vi "testTwoServersReportLogMessages.vi"(8 "error in":errorcluster) -> (0 "error out":errorcluster)   [LabVIEW 2018]
uses:
  <vilib>/addons/_JKI Toolkits/Caraya/classes/Assert/Assert Equal Value_Variant.vi
  <vilib>/addons/_JKI Toolkits/Caraya/classes/Test/Test.lvclass
  <vilib>/addons/_JKI Toolkits/Caraya/classes/Assert/Assert.lvclass
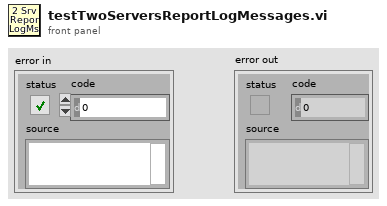
[diagram p1: front panel]
types:
  T1 = cluster{"CmdRead":refnum<user-event>, "EvtRead":refnum<user-event>, "GenRead":refnum<user-event>}
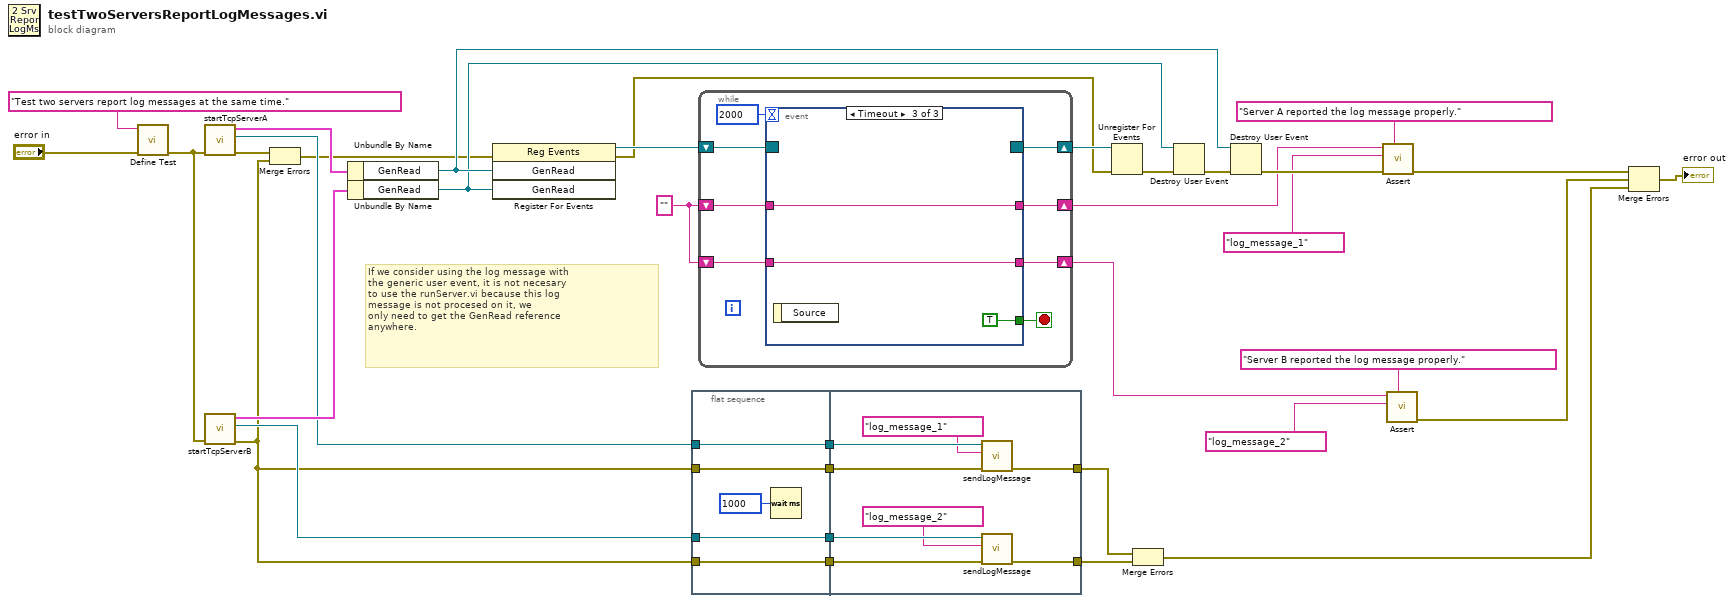
[diagram p0: block diagram]
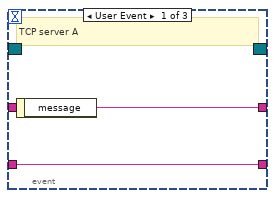
[diagram p2: hidden frame]
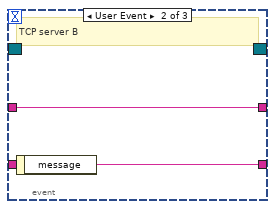
[diagram p3: hidden frame]
diagram:
  w7 = ""
  # "If we consider using the log message with\nthe generic user event, it is not necesary\nto use the runServer.vi because this log\nmessage is not procesed on it, we\nonly need to get the GenRead reference\nanywhere."
  # "Event Structure for TCP server B"
  # "Event Structure for TCP server A"
  n1 = call <vilib>:"Define Test.vi"("error in (no error)"="error in", "Label (VI Title)"="Test two servers report log messages at the same time.") -> ("error out"=w33:errorcluster)  [unwired: 9 in]
  n2 = call "startTcpServerA.vi"("error in (no error)"=w33) -> ("error out"=w21:errorcluster, "TcpServer out"=w15:refnum<class "TcpServer.lvclass">, "UserEvents"=w32:T1)  [unwired: 8 in]
  n3 = call "startTcpServerB.vi"("error in (no error)"=w33) -> ("error out"=w1:errorcluster, "TcpServer out"=w12:refnum<class "TcpServer.lvclass">, "UserEvents"=w31:T1)  [unwired: 8 in]
  n4 = Merge Errors(w21, w1) -> (w2:errorcluster)
  n5 = Unbundle By Name(w32) -> ("GenRead"=w24:refnum<user-event>)
  n6 = Unbundle By Name(w31) -> ("GenRead"=w8:refnum<user-event>)
  n7 = register-events(error in=w2, w24, w8) -> (reference out=w30:refnum<event-registration>, error out=w20:errorcluster)  [unwired: 1 in]
  n8 = flat-sequence {
    tunnel: [w40] -> w29
    tunnel: [w39] -> w14
    tunnel: [w38] -> w13
    tunnel: w12 -> [w38]
    tunnel: w15 -> [w39]
    tunnel: w1 -> [w40]
    tunnel: w1 -> [w36]
    tunnel: [w36] -> w11
    tunnel: [w48] -> w27
    tunnel: [w47] -> w26
    tunnel: w11 -> [w41]
    tunnel: w13 -> [w44]
    tunnel: w14 -> [w45]
    tunnel: w29 -> [w46]
    frame #0 {
      n9 = Wait (ms)(milliseconds to wait=u32 1000) -> ()  [unwired: 1 out]
    }
    frame #1 {
      n10 = call "sendLogMessage.vi"("error in (no error)"=w46, "message"="log_message_1", "tcpServer in"=w45) -> ("error out"=w48:errorcluster)  [unwired: 7 in, 1 out]
      n11 = call "sendLogMessage.vi"("error in (no error)"=w41, "message"="log_message_2", "tcpServer in"=w44) -> ("error out"=w47:errorcluster)  [unwired: 7 in, 1 out]
    }
  }
  n12 = while {
    shift-right: [w55] -> w28
    shift-left: w30 -> [w56]
    shift-right: [w54] -> w6
    shift-left: w7 -> [w53]
    shift-right: [w49] -> w4
    shift-left: w7 -> [w52]
    stop <- w50 stop-if-true
    n13 = event shown="[2] Timeout" {
      selector: w56 -> [_ _ _]
      dyn-events: [_ _ _] -> w55
      timeout: 2000 -> [_ _ _]
      tunnel: [w58 w60 w62] -> w54
      tunnel: w53 -> [_ w60 w62]
      tunnel: [w57 w59 w61] -> w49
      tunnel: w52 -> [w57 _ w61]
      tunnel: [_ _ TRUE] -> w50
      event User Event {
        # "TCP server A"
        n14 = event-data() -> ("message"=w58:string)  [unwired: 1 in]
      }
      event User Event {
        # "TCP server B"
        n15 = event-data() -> ("message"=w59:string)  [unwired: 1 in]
      }
      event Timeout {
        n16 = event-data() -> ()  [unwired: 1 in, 1 out]
      }
    }
  }
  n17 = Unregister For Events(event registration refnum=w28, error in=w20) -> (error out=w9:errorcluster)
  n18 = Merge Errors(w27, w26) -> (w25:errorcluster)
  n19 = Destroy User Event(user event=w8, error in=w9) -> (error out=w10:errorcluster)
  n20 = Destroy User Event(user event=w24, error in=w10) -> (error out=w19:errorcluster)
  n21 = call-poly <vilib>:"Assert.vi"("Label"="Server A reported the log message properly.", "error in (no error)"=w19, "Y"="log_message_1", "X"=w6) -> ("error out"=w16:errorcluster)  [unwired: 7 in]
  n22 = call-poly <vilib>:"Assert.vi"("Label"="Server B reported the log message properly.", "Y"="log_message_2", "X"=w4) -> ("error out"=w17:errorcluster)  [unwired: 8 in]
  n23 = Merge Errors(w16, w17, w25) -> (→"error out":errorcluster)
